vi "1 Tap 16-Bit.vi"() -> (0 "Pixels":cluster{"Pixel 0":u16})   [LabVIEW 2014]
uses:
  <vilib>/rvi/eio/common/nirviEmuTemplateMethod_errors.vi
  <vilib>/eio/EIONode/EIONode.xnode
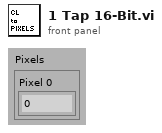
[diagram p1: front panel]
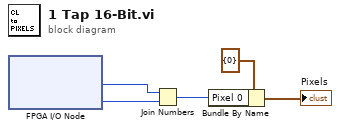
[diagram p0: block diagram]
diagram:
  n1 = xnode "FPGA I/O Node"() -> ("CL Port B"=w4:u8, "CL Port A"=w5:u8)  [unwired: 2 in, 2 out]
  n2 = Join Numbers(hi=w4, lo=w5) -> ((hi.lo)=w3:u16)
  n3 = Bundle By Name(cluster=cluster{"Pixel 0":u16} {"Pixel 0"=0} ("Data"), "Pixel 0"=w3) -> (→"Pixels":cluster{"Pixel 0":u16})
